vi "计算二阶正图像.vi"(0 "关联成像原理":dbl, 5 "重建方法":dbl, 7 "光源散斑簇":T1, 9 "差分计算一维矩阵":dbl[](array[numeric]), 11 "正图像筛选门限":dbl) -> (4 "未归一化二阶正图像":dbl[][](array[numeric]))   [LabVIEW 2018]
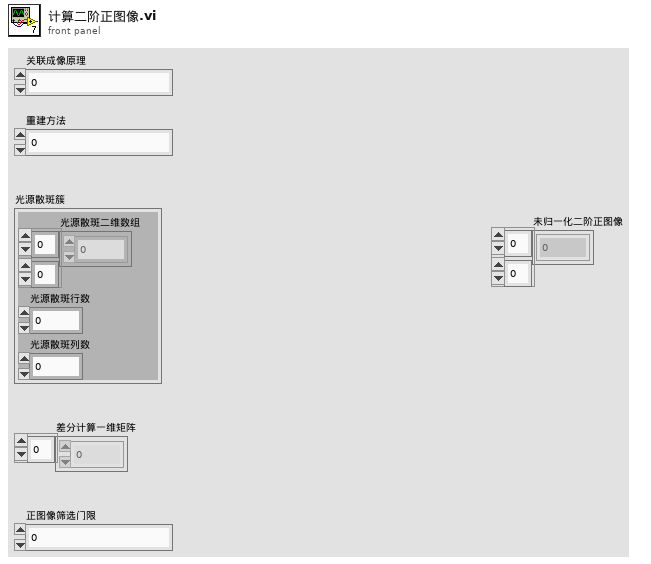
[diagram p1: front panel]
types:
  T1 = cluster{"光源散斑二维数组":dbl[][], "光源散斑行数":i32, "光源散斑列数":i32}
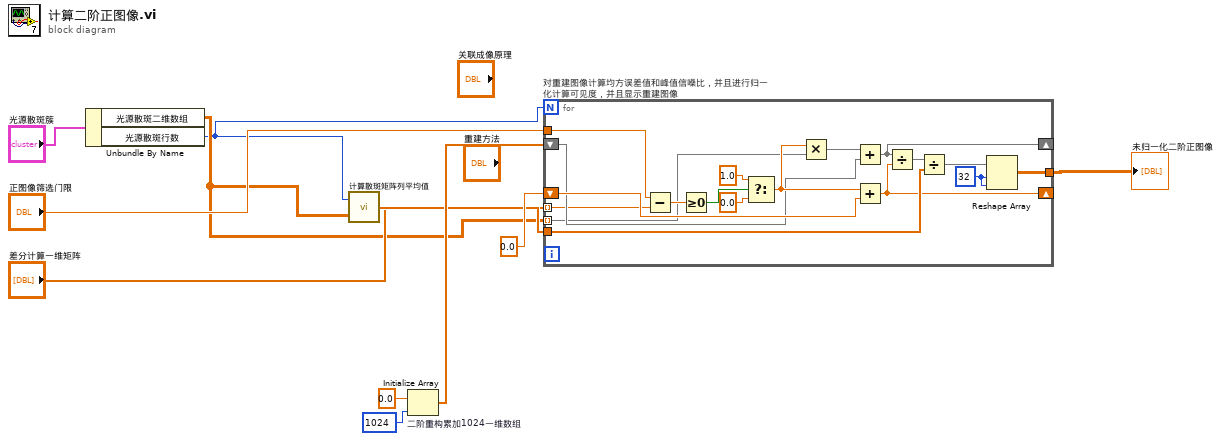
[diagram p0: block diagram]
diagram:
  n1 = Unbundle By Name("光源散斑簇") -> ("光源散斑二维数组"=w2:dbl[][], "光源散斑行数"=w1:i32)
  n2 = call "计算散斑矩阵列平均值.vi"("散斑二维数组"=w2, "散斑二维数组行数"=w1) -> ("散斑二维数组列平均值"=w5:dbl[])
  n3 = Initialize Array "二阶重构累加1024一维数组"(0.0 ("元素"), 1024 ("维数大小")) -> (w7:dbl[])
  n4 = for "对重建图像计算均方误差值和峰值信噪比，并且进行归一化计算可见度，并且显示重建图像" {
    N: w1 -> [_]
    tunnel: w2 -> [w13] mode=indexing
    shift-right: [w17] -> _
    shift-left: w7 -> [w16]
    shift-right: [w15] -> _
    shift-left: 0.0 ("数值") -> [w23]
    tunnel: "正图像筛选门限" -> [w29]
    tunnel: w5 -> [w18]
    tunnel: [w14] -> w6
    tunnel: "差分计算一维矩阵" -> [w12] mode=indexing
    w22 = 32 ("维数大小")
    n5 = Subtract(x=w29, y=w12) -> (x-y=w25:dbl)
    n6 = Greater Or Equal To 0?(x=w25) -> (x >= 0?=w28:bool)
    n7 = Select(t=1.0, s=w28, f=0.0) -> (s? t:f=w24:dbl)
    n8 = Multiply(x=w24, y=w13) -> (x*y=w19:dbl[])
    n9 = Add(x=w19, y=w16) -> (x+y=w17:dbl[])
    n10 = Add(x=w24, y=w23) -> (x+y=w15:dbl)
    n11 = Divide(x=w17, y=w15) -> (x/y=w21:dbl[])
    n12 = Divide(x=w21, y=w18) -> (x/y=w20:dbl[])
    n13 = Reshape Array(w20, w22, w22) -> (w14:dbl[][])
  }
  "未归一化二阶正图像" <- w6
